vi "2_2_PatchCore_Inference(Camera)(Snap).vi"() -> ()   [LabVIEW 2024]
uses:
  <vilib>/Ngene/DeepLTK Anomaly Detection Addon/DeepLTK_Anomaly_Detection_Addon/API/Controls/NN_Paths.ctl
  <vilib>/Ngene/Deep Learning Toolkit/Toolkit/NN_Data/API/NN_Dims(C,H,W).ctl
  <vilib>/Ngene/Deep Learning Toolkit/Toolkit/NN_Network/Controls/NN_Device.ctl
  subVIs/Visualizer/Controls/Display_Options.ctl
  subVIs/Visualizer/Controls/ROI_Display_Options.ctl
  subVIs/Visualizer/Controls/Heatmap_Display_Options.ctl
  subVIs/Visualizer/Controls/ColorMap.ctl
  <vilib>/Ngene/DeepLTK Anomaly Detection Addon/DeepLTK_Anomaly_Detection_Addon/API/Controls/MinMax.ctl
  subVIs/Camera/Controls/Camera_Settings.ctl
  <vilib>/vision/driver/IMAQdx.llb/IMAQdx Acquisition Mode.ctl
  <vilib>/vision/driver/IMAQdx.llb/IMAQdx Camera Control Mode.ctl
  <vilib>/Ngene/DeepLTK Anomaly Detection Addon/DeepLTK_Anomaly_Detection_Addon/API/Controls/NNPC_Setup.ctl
  <vilib>/vision/driver/IMAQdx.llb/IMAQdx Buffer Number Mode.ctl
  <vilib>/Ngene/DeepLTK Anomaly Detection Addon/DeepLTK_Anomaly_Detection_Addon/API/Controls/Feature_Scorer_Params.ctl
  <vilib>/Ngene/DeepLTK Anomaly Detection Addon/DeepLTK_Anomaly_Detection_Addon/API/Controls/Gaussian_Blur.ctl
  <vilib>/Ngene/DeepLTK Anomaly Detection Addon/DeepLTK_Anomaly_Detection_Addon/API/NNPC_Predict/NNPC_Predict(Single).vi
  <vilib>/Ngene/DeepLTK Anomaly Detection Addon/DeepLTK_Anomaly_Detection_Addon/DeepLTK_Anomaly_Detection_Addon.lvlib
  <vilib>/ptbypt/NI_PtbyPt.lvlib
  <vilib>/vision/driver/NI_Vision_Acquisition_Software.lvlib
  <vilib>/Ngene/Deep Learning Toolkit/Toolkit/Deep_Learning_Toolkit_by_Ngene.lvlib
panel:
  in  "Tab Control 2":enum32{"CFG", "Demo"}(tab)
  out "dT_Forward":dbl=0.5810284729999466 format="%#_3p"
  in  "Stop":bool
  out "Dims_In":T1={"C"=3, "H"=224, "W"=224}
  out "Loop Time":dbl=0.8034906005000266 format="%.2ps"
  out "Preproc. Time":dbl=0.010750834499958728 format="%.2ps"
  in  "Image_Thrshld":sgl=-1.0 format="%_5g"
  out "Pixel_Score(Max)":sgl=14.516328
  out "Img_Score":sgl=14.816199
  in  "Pixel_Thrshld":sgl=8.400001 format="%_5g"
  out "Error Count":i16
  in  "Camera_Settings":T2={"Camera_Resolution"=203, "Focus"=35, "Exposure"=5, "Gain"=50, "WhiteB."=6457} {"WhiteB." min=2000 max=7500 step=1; "Gain" max=255 step=1; "Exposure" min=0 max=9 step=1; "Focus" step=5}
  in  "Rel Margin":sgl=0.02
  in  "Camera":refnum<k21>="cam2" caption="IMAQdx Session"
  in  "Display_Options":T3={"ROI_Options"={"Color"=16711713, "Width"=4, "Drawing Mode"=enum."Frame"}, "Heatmap_Options"={"ColorMap"=enum."Jet", "Alpha"=0.4, "Heatmap Range"={"Min"=8.0, "Max"=-1.0}}, "Has GT?"=FALSE} {"Heatmap_Options"."Heatmap Range"."Min" format="%#_5g"}
  in  "Trained_Model_Paths":T8={"CFG"=path "D:/Ngene/GitHub/niconnect2025/VAD_Card_RT_v2.0_vad2.1/Models/3_Clubs_Demo_v2/NNPC_3Clubs__25_04_23__20_03_43_Fast/NNPC_3Clubs.cfg", "BIN"=path "D:/Ngene/GitHub/niconnect2025/VAD_Card_RT_v2.0_vad2.1/Models/3_Clubs_Demo_v2/NNPC_3Clubs__25_04_23__20_03_43_Fast/NNPC_3Clubs.bin"}
  in  "Device":T9
  in  "Center_Crop_Size":i32=680
  out "Prediction":bool=TRUE
  out "Device Name":string="sbRIO-9609"
  out "Inference Time":dbl=0.7674025689999553 format="%_3ps"
  out "FPS":dbl=1.3030970189520674 format="%.2f"
  out "Anomaly Detection Results":T10(plugin-control)
  # "Unsupervised \nVisual Anomaly Detection"
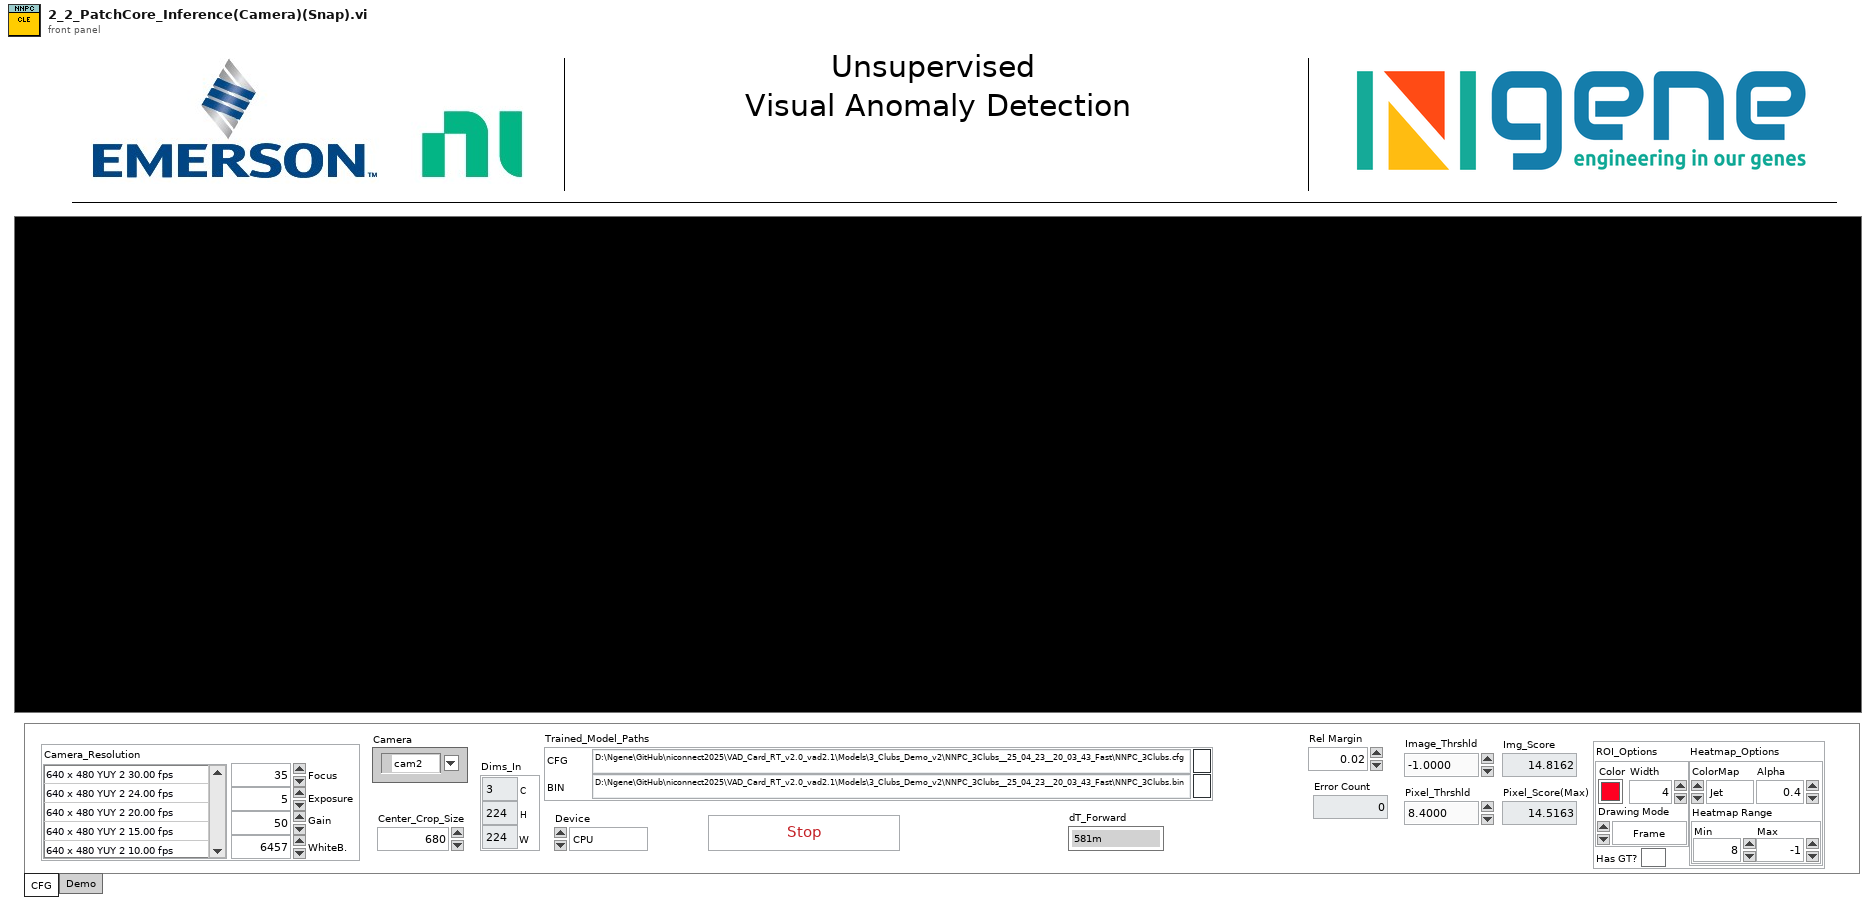
[diagram p1: front panel]
types:
  T1 = typedef "Deep_Learning_Toolkit_by_Ngene.lvlib/NN_Dims(C,H,W).ctl" = cluster{"C":i32, "H":i32, "W":i32}
  T2 = typedef "Camera_Settings.ctl" = cluster{"Camera_Resolution":i32, "Focus":u8, "Exposure":i32, "Gain":u32, "WhiteB.":i32}
  T3 = typedef "Display_Options.ctl" = cluster{"ROI_Options":T4, "Heatmap_Options":T5, "Has GT?":bool}
  T4 = typedef "ROI_Display_Options.ctl" = cluster{"Color":u32, "Width":u32, "Drawing Mode":enum16{"Frame", "Fill"}}
  T5 = typedef "Heatmap_Display_Options.ctl" = cluster{"ColorMap":T6, "Alpha":sgl, "Heatmap Range":T7}
  T6 = typedef "ColorMap.ctl" = enum16{"Jet", "Perula", "Inferno", "Plasma", "Viridis"}
  T7 = typedef "DeepLTK_Anomaly_Detection_Addon.lvlib/MinMax.ctl" = cluster{"Min":sgl, "Max":sgl}
  T8 = typedef "DeepLTK_Anomaly_Detection_Addon.lvlib/NN_Paths.ctl" = cluster{"CFG":path, "BIN":path}
  T9 = typedef "Deep_Learning_Toolkit_by_Ngene.lvlib/NN_Device.ctl" = enum16{"CPU", "GPU"}
  T10 = typedef "IMAQ Image.ctl" = refnum<image>
  T11 = typedef "NI_Vision_Acquisition_Software.lvlib/IMAQdx Acquisition Mode.ctl" = enum32{"One Shot", "Continuous"}
  T12 = typedef "Image Type" = u32
  T13 = typedef "NI_Vision_Acquisition_Software.lvlib/IMAQdx Camera Control Mode.ctl" = enum32{"Controller", "Listener"}
  T14 = typedef "DeepLTK_Anomaly_Detection_Addon.lvlib/NNPC_Setup.ctl" = cluster{"Input_Dims":T1, "mBatch":i32, "Device":T9, "GPU Id":i32}
  T15 = typedef "IMAQdx.ctl" = refnum<k21>
  T16 = typedef "DeepLTK_Anomaly_Detection_Addon.lvlib/NNPC_Evaluation_Results.ctl" = cluster{"Threshold(Image)":sgl, "Threshold(Pixel)":sgl, "Pixel_Range":cluster{"Min":sgl, "Max":sgl}}
  T17 = typedef "DeepLTK_Anomaly_Detection_Addon.lvlib/NNPC_PreProcessing_Options.ctl" = cluster{"DS_Name":string, "Input_Dims":T1, "Center Crop Size":i32, "Interpolation Type":u32, "Multi-Stage_DownSample?":bool, "Dataset_Stats":T18}
  T18 = typedef "DeepLTK_Anomaly_Detection_Addon.lvlib/NNPC_DS_Stats.ctl" = cluster{"means":T19, "stds":T19}
  T19 = typedef "DeepLTK_Anomaly_Detection_Addon.lvlib/Image_Stats_RGB.ctl" = cluster{"R":sgl, "G":sgl, "B":sgl}
  T20 = typedef "DeepLTK_Anomaly_Detection_Addon.lvlib/NNPC_Instance.ctl" = cluster{"NN out":T21, "MemBank_Data":T36, "Name":string}
  T21 = typedef "Deep_Learning_Toolkit_by_Ngene.lvlib/NN.ctl" = cluster{"Name":string, "No of Layers":i32, "mBatch":i32, "Layers":T22[], "Dimty":T23, "Dims_In":T1, "Dims_Out":T1, "Working_Dir":path, "Train?":bool, "Train_Params":T24, "LR_Update_Policy":T27, "Session Data":T29, "Ground_truth":T30, "NNg_hdls":T31, "NN_Device":T9, "GPU Id":i32, "Labels":string[], "Receptive Field":T32[], "Loss_Type":T33, "Loss_Cfg_Prms":variant, "NNG_WS":T34}
  T22 = typedef "Deep_Learning_Toolkit_by_Ngene.lvlib/NN_Layer_ref.ctl" = refnum<data-value>
  T23 = typedef "Deep_Learning_Toolkit_by_Ngene.lvlib/NN_In_Out_Dim-ty.ctl" = enum8{"In1D_Out1D", "In3D_Out1D", "In3D_Out3D", "In3D_OutBBox"}
  T24 = typedef "Deep_Learning_Toolkit_by_Ngene.lvlib/NN_Train_Params.ctl" = cluster{"Optimizer":T25, "Beta_1":sgl, "Beta_2":sgl, "Weight Decay(L1)":sgl, "Weight Decay(L2)":sgl, "Data_Sampling":T26}
  T25 = typedef "Deep_Learning_Toolkit_by_Ngene.lvlib/NN_Train_Optimizer.ctl" = enum16{"SGD", "Adam", "Adagrad", "Adadelta", "RMSProp", "Nesterov"}
  T26 = typedef "Deep_Learning_Toolkit_by_Ngene.lvlib/NN_Train_Data_Sampling.ctl" = enum16{"Random", "Sequential"}
  T27 = typedef "Deep_Learning_Toolkit_by_Ngene.lvlib/NN_LR_Policy_Cfg.ctl" = cluster{"Policy_Type":T28, "LR0":dbl, "k":sgl, "WarmUp_Policy":enum16{"Step", "Ramp"}, "WarmUp_Iter":i32, "WarmUp_Ratio":sgl}
  T28 = typedef "Deep_Learning_Toolkit_by_Ngene.lvlib/NN_LR_Policy_Type.ctl" = enum16{"Manual", "Step", "Exp", "1/t"}
  T29 = typedef "Deep_Learning_Toolkit_by_Ngene.lvlib/NN_Train_Session_Data.ctl" = cluster{"Epochs":sgl, "Tot_Iter":i32, "LR":sgl, "LR_iter":i32}
  T30 = typedef "Deep_Learning_Toolkit_by_Ngene.lvlib/NN_Ground_truth.ctl" = cluster{"Y":variant}
  T31 = typedef "Deep_Learning_Toolkit_by_Ngene.lvlib/nng_cuda_handles.ctl" = cluster{"cudnn":u64, "cublas":u64, "stream":u64, "curand":u64}
  T32 = typedef "Deep_Learning_Toolkit_by_Ngene.lvlib/NN_Dims(V,H).ctl" = cluster{"V":i32, "H":i32}
  T33 = typedef "Deep_Learning_Toolkit_by_Ngene.lvlib/NN_Loss_Type.ctl" = enum16{"None", "MSE", "CrossEntropy", "YOLO_v2", "YOLO_v4"}
  T34 = typedef "Deep_Learning_Toolkit_by_Ngene.lvlib/NNG_WS.ctl" = cluster{"NNG_WS_Mem":T35, "Max_WS_Size":i64}
  T35 = typedef "Deep_Learning_Toolkit_by_Ngene.lvlib/NNg_WS_Mem_DVR.ctl" = refnum<data-value>
  T36 = typedef "DeepLTK_Anomaly_Detection_Addon.lvlib/MemBank_and_Norm_Variants.ctl" = cluster{"MemBank":variant, "MemBank Norm":variant}
  T37 = typedef "NI_Vision_Acquisition_Software.lvlib/IMAQdx Buffer Number Mode.ctl" = enum32{"Next", "Last", "Buffer Number", "Every", "Last New"}
  T38 = typedef "DeepLTK_Anomaly_Detection_Addon.lvlib/Feature_Scorer_Params.ctl" = cluster{"Nearest_Neighbors":i32, "Calculate Anomaly Map":bool, "Gaussian_Blur":T39}
  T39 = typedef "DeepLTK_Anomaly_Detection_Addon.lvlib/Gaussian_Blur.ctl" = cluster{"Kernel_Size":i32, "Sigma":sgl}
  T40 = typedef "Anomaly_Detection_Results_Imgs.ctl" = cluster{"Image":T10, "Ground Truth":T10, "Predicted Heat Map":T10, "Predicted Mask":T10, "Segmentation":T10}
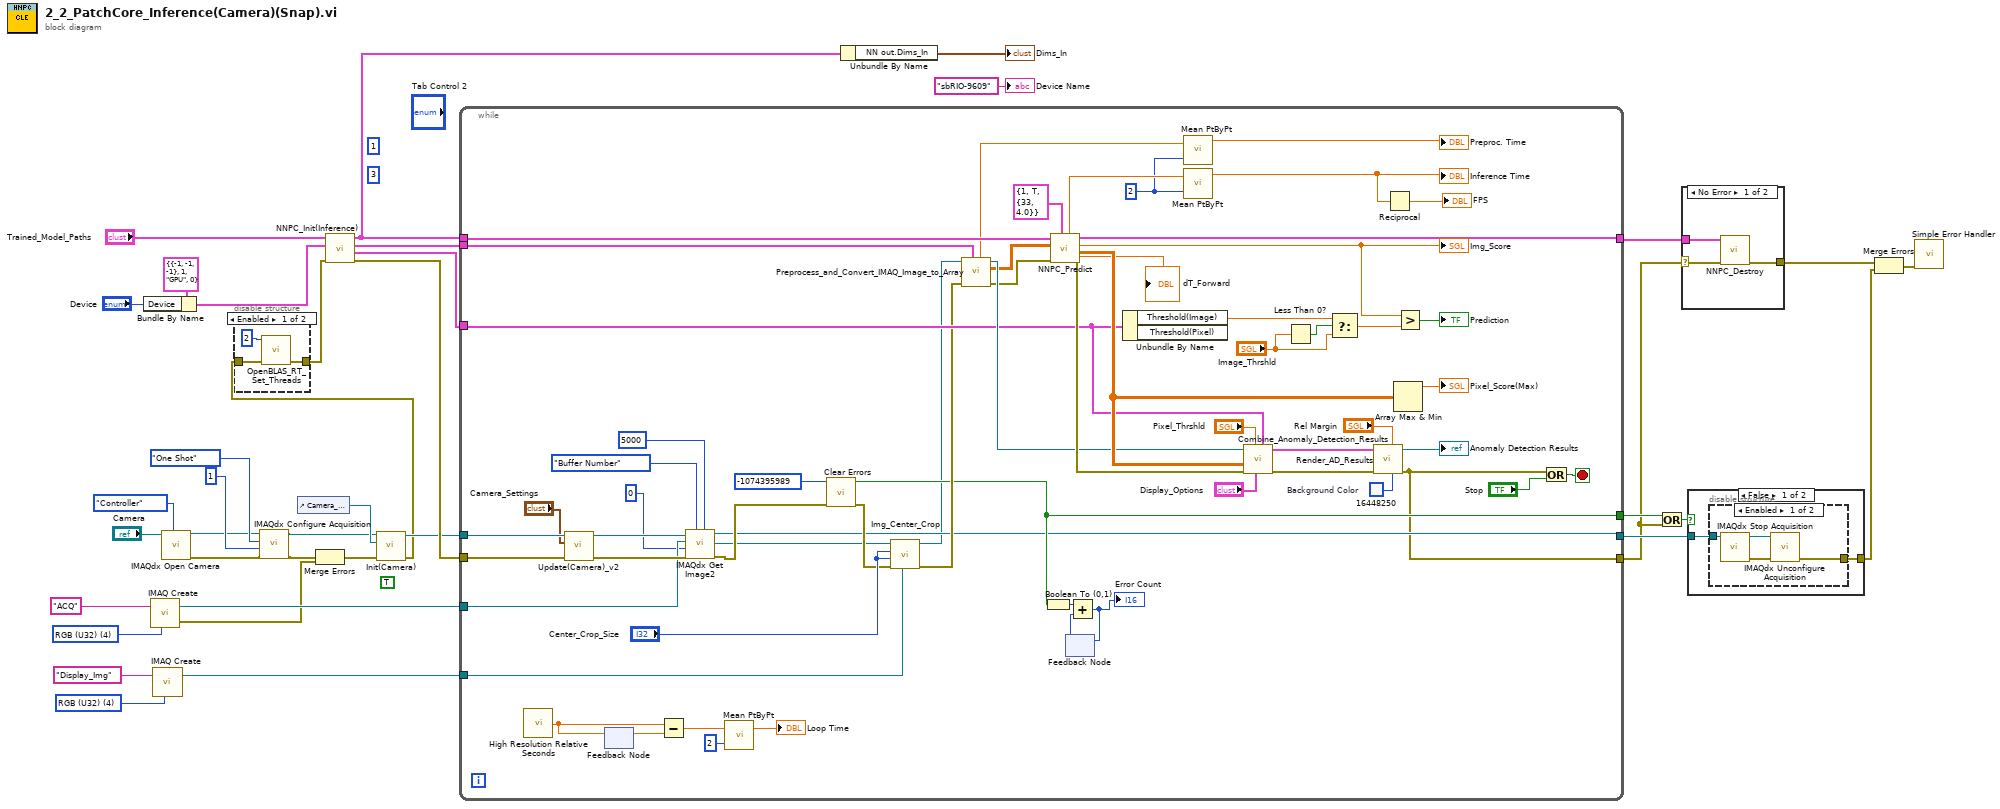
[diagram p0: block diagram]
diagram:
  (unwired) TRUE
  (unwired) i64 1 ("Period")
  (unwired) 3 ("Processor")
  w15 = T12 4 items=["Grayscale (U8)", "Grayscale (I16)", "Grayscale (SGL)", "Complex (CSG)", "RGB (U32)", "HSL (U32)", "RGB (U64)", "Grayscale (U16)"] ("Image Type")
  w24 = T12 4 items=["Grayscale (U8)", "Grayscale (I16)", "Grayscale (SGL)", "Complex (CSG)", "RGB (U32)", "HSL (U32)", "RGB (U64)", "Grayscale (U16)"] ("Image Type")
  n1 = Bundle By Name(cluster=T14 {"Input_Dims"={"C"=-1, "H"=-1, "W"=-1}, "mBatch"=1, "Device"=enum."GPU", "GPU Id"=0} ("NNFE_CFG"), "Device"="Device") -> (w20:T14)
  n2 = call "IMAQ Create"("Image Name"="ACQ", "Image Type"=w24) -> ("New Image"=w21:T10, "error out"=w18:errorcluster)  [unwired: 3 in]
  n3 = call "IMAQ Create"("Image Name"="Display_Img", "Image Type"=w15) -> ("New Image"=w13:T10)  [unwired: 3 in, 1 out]
  n4 = call <vilib>:"IMAQdx Open Camera.vi"("Camera Control Mode"=IMAQdx_Camera_Control_Mode."Controller", "Session In"="Camera") -> ("error out"=w5:errorcluster, "Session Out"=w1:T15)  [unwired: 1 in, 7 out]
  n5 = call <vilib>:"IMAQdx Configure Acquisition.vi"("error in"=w5, "Number of Buffers"=u32 1, "Continuous?"=IMAQdx_Acquisition_Mode."One Shot", "Session In"=w1) -> ("error out"=w4:errorcluster, "Session Out"=w6:T15)  [unwired: 6 in]
  n6 = control-ref of="Camera_Settings"() -> (w19:refnum<vi>)
  n7 = Merge Errors(w4, w18) -> (w22:errorcluster)
  n8 = call "Init(Camera).vi"("error in (no error)"=w22, "Camera_Settings_Ref"=w19, "Session in"=w6) -> ("error out"=w7:errorcluster, "Session out"=w8:T15)  [unwired: 7 in]
  n9 = disable-structure shown="Enabled" {
    disable-tunnel: [w41 _] -> w16
    disable-tunnel: w7 -> [w39 _]
    frame Enabled {
      n10 = call "OpenBLAS_RT_Set_Threads.vi"("error in (no error)"=w39, "threads"=2) -> ("error out"=w41:errorcluster)  [unwired: 9 in]
    }
    frame Disabled {
    }
  }
  n11 = call <vilib>:"NNPC_Init(Inference).vi"("error in"=w16, "NNPC_Setup"=w20, "NNPC_Paths"="Trained_Model_Paths") -> ("error out"=w9:errorcluster, "Evaluation_Results"=w34:T16, "PreProc_Options"=w35:T17, "NNPC_out"=w30:T20)  [unwired: 4 in, 1 out]
  n12 = while {
    tunnel: w30 -> [w92]
    tunnel: [w87] -> w38
    tunnel: w35 -> [w79]
    tunnel: w34 -> [w74]
    tunnel: [w51] -> w33
    tunnel: [w50] -> w10
    tunnel: w9 -> [w67]
    tunnel: w8 -> [w70]
    tunnel: w21 -> [w66]
    tunnel: w13 -> [w57]
    tunnel: [w54] -> w12
    stop <- w86 stop-if-true
    w49 = 2 ("sample length")
    w85 = u32 16448250  # Background Color
    n13 = call <vilib>:"High Resolution Relative Seconds.vi"() -> ("relative seconds"=w81:dbl)
    n14 = call "Update(Camera)_v2.vi"("error in (no error)"=w67, "Camera_Settings"="Camera_Settings", "Session in"=w70) -> ("error out"=w69:errorcluster, "Session out"=w68:T15)  [unwired: 7 in]
    n15 = feedback #1() -> (w82:dbl)  [unwired: 1 in]
    n16 = feedback-in #1(w81) -> ()
    n17 = Subtract(x=w81, y=w82) -> (x-y=w80:dbl)
    n18 = call <vilib>:"IMAQdx Get Image2.vi"("Timeout (ms)"=5000, "Buffer Number Mode (Next)"=IMAQdx_Buffer_Number_Mode."Buffer Number" ("Buffer Number Mode"), "error in"=w69, "Buffer Number In"=u32 0, "Image In"=w66, "Session In"=w68) -> ("error out"=w59:errorcluster, "Image Out"=w58:T10, "Session Out"=w51:T15)  [unwired: 2 in, 1 out]
    n19 = call <vilib>:"Mean PtByPt.vi"("x"=w80, "sample length"=2) -> ("mean"=→"Loop Time":dbl)  [unwired: 2 in, 1 out]
    n20 = call <vilib>:"Clear Errors.vi"("error in (no error)"=w59, "specific error code to clear (0: all)"=-1074395989) -> ("error out"=w61:errorcluster, "specific error cleared?"=w54:bool)  [unwired: 4 in]
    n21 = call "Img_Center_Crop.vi"("Image Dst"=w57, "error in (no error)"=w61, "height"="Center_Crop_Size", "width"="Center_Crop_Size", "Image In"=w58) -> ("error out"=w63:errorcluster, "Image Out"=w45:T10)  [unwired: 5 in]
    n22 = call "Preprocess_and_Convert_IMAQ_Image_to_Array.vi"("PreProcessing_Options"=w79, "error in (no error)"=w63, "Imaq Image In"=w45) -> ("error out"=w75:errorcluster, "Norm_Img_Out"=w62:sgl[][][], "Imaq Image Out"=w76:T10, "dT_Preprocessing"=w77:dbl)  [unwired: 5 in]
    n23 = Boolean To (0,1)(Boolean=w54) -> (0, 1=w53:i16)
    n24 = call-poly <vilib>:"NNPC_Predict.vi"("Feature_Scorer_Params"=T38 {"Nearest_Neighbors"=1, "Calculate Anomaly Map"=TRUE, "Gaussian_Blur"={"Kernel_Size"=33, "Sigma"=4.0}}, "error in"=w75, "Image_in"=w62, "NNPC_in"=w92) -> ("error out"=w102:errorcluster, "Anomaly_Map"=w91:sgl[][], "Pred_Score"=w90:sgl, "NNPC_out"=w87:T20, "dT_Forward"=→"dT_Forward":dbl, "dT_Predict"=w84:dbl)  [unwired: 2 in]
    "Img_Score" <- w90
    n25 = feedback #2() -> (w55:i16)  [unwired: 1 in]
    n26 = Add(x=w53, y=w55) -> (x+y=w52:i16)
    "Error Count" <- w52
    n27 = feedback-in #2(w52) -> ()
    n28 = Unbundle By Name(w74) -> ("Threshold(Image)"=w83:sgl)  [unwired: 1 out]
    n29 = call <vilib>:"Mean PtByPt.vi"("x"=w77, "sample length"=w49) -> ("mean"=→"Preproc. Time":dbl)  [unwired: 2 in, 1 out]
    n30 = call <vilib>:"Mean PtByPt.vi"("x"=w84, "sample length"=w49) -> ("mean"=w48:dbl)  [unwired: 2 in, 1 out]
    "Inference Time" <- w48
    n31 = call "Combine_Anomaly_Detection_Results.vi"("Evaluation_Results"=w74, "Display_Options"="Display_Options", "Pixel Anomaly Thrshld"="Pixel_Thrshld", "error in"=w102, "Anomaly Map"=w91, "Orig Image In"=w76) -> ("error out"=w101:errorcluster, "Anomaly Detection Rresults"=w100:T40)  [unwired: 3 in, 1 out]
    n32 = Less Than 0?(x="Image_Thrshld") -> (x < 0?=w96:bool)
    n33 = Select(t=w83, s=w96, f="Image_Thrshld") -> (s? t:f=w94:sgl)
    n34 = call "Render_AD_Results.vi"("Background Color"=w85, "Rel._Margin"="Rel Margin", "error in"=w101, "Anomaly Detection Rresults"=w100) -> ("error out"=w50:errorcluster, "Anomaly Detection Results"=→"Anomaly Detection Results":T10)  [unwired: 6 in]
    n35 = Reciprocal(x=w48) -> (1/x=→"FPS":dbl)
    n36 = Array Max & Min(array=w91) -> (max value=→"Pixel_Score(Max)":sgl)  [unwired: 3 out]
    n37 = Greater?(x=w90, y=w94) -> (0:→"Prediction":bool)
    n38 = Or(x=w50, y="Stop") -> (x .or. y?=w86:bool)
  }
  n39 = Unbundle By Name(w30) -> ("NN out.Dims_In"=→"Dims_In":T1)
  n40 = Or(x=w12, y=w10) -> (x .or. y?=w11:bool)
  n41 = case shown="No Error" w10 {
    selector: w10 -> [w103 w106]
    tunnel: w38 -> [w105 _]
    tunnel: [w104 w106] -> w37
    frame No Error {
      n42 = call <vilib>:"NNPC_Destroy.vi"("error in"=w103, "NNPC_in"=w105) -> ("error out"=w104:errorcluster)  [unwired: 9 in]
    }
    frame Error {
    }
  }
  n43 = case shown="False" w11 {
    tunnel: w33 -> [w108 _]
    tunnel: [w107 _] -> w31
    frame False {
      n44 = disable-structure shown="Enabled" {
        disable-tunnel: w108 -> [w112 _]
        disable-tunnel: [w109 _] -> w107
        frame Enabled {
          n45 = call <vilib>:"IMAQdx Stop Acquisition.vi"("Session In"=w112) -> ("error out"=w110:errorcluster, "Session Out"=w111:T15)  [unwired: 9 in]
          n46 = call <vilib>:"IMAQdx Unconfigure Acquisition.vi"("error in"=w110, "Session In"=w111) -> ("error out"=w109:errorcluster)  [unwired: 8 in, 1 out]
        }
        frame Disabled {
        }
      }
    }
    frame True {
    }
  }
  n47 = Merge Errors(w37, w31) -> (w32:errorcluster)
  n48 = call <vilib>:"Simple Error Handler.vi"("error in (no error)"=w32) -> ()  [unwired: 4 in, 5 out]
  "Device Name" <- "sbRIO-9609" ("Device Name")
